vi "Inclinometer_DataTranslation.vi"(11 "read buffer":string) -> (3 "X Axis":dbl)   [LabVIEW 2019]
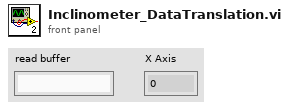
[diagram p1: front panel]
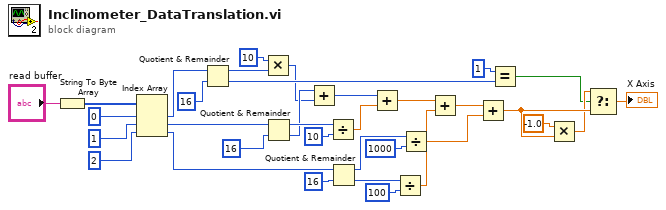
[diagram p0: block diagram]
diagram:
  n1 = String To Byte Array(string="read buffer") -> (unsigned byte array=w2:u8[])
  n2 = Index Array(array=w2, index #1=0 ("index"), index #2=1 ("index"), index #3=2 ("index")) -> (element #1=w6:u8, element #2=w8:u8, element #3=w10:u8)
  n3 = Quotient & Remainder(x=w6, y=u8 16) -> (x-y*floor(x/y)=w14:u8, floor(x/y)=w28:u8)
  n4 = Multiply(x=u8 10, y=w14) -> (x*y=w13:u8)
  n5 = Quotient & Remainder(x=w8, y=u8 16) -> (x-y*floor(x/y)=w17:u8, floor(x/y)=w15:u8)
  n6 = Add(x=w15, y=w13) -> (x+y=w16:u8)
  n7 = Divide(x=w17, y=u8 10) -> (x/y=w19:dbl)
  n8 = Quotient & Remainder(x=w10, y=u8 16) -> (x-y*floor(x/y)=w25:u8, floor(x/y)=w21:u8)
  n9 = Add(x=w16, y=w19) -> (x+y=w22:dbl)
  n10 = Divide(x=w21, y=u8 100) -> (x/y=w23:dbl)
  n11 = Divide(x=w25, y=u16 1000) -> (x/y=w27:dbl)
  n12 = Add(x=w22, y=w23) -> (x+y=w26:dbl)
  n13 = Add(x=w26, y=w27) -> (x+y=w33:dbl)
  n14 = Equal?(x=u8 1, y=w28) -> (x = y?=w30:bool)
  n15 = Multiply(x=-1.0, y=w33) -> (x*y=w32:dbl)
  n16 = Select(t=w32, s=w30, f=w33) -> (s? t:f=→"X Axis":dbl)
